vi "User Message Received.vi"(0 "Member in":refnum<class "Member.lvclass">, 5 "Message":refnum<class "Message.lvclass">, 11 "Error in":errorcluster caption="Error in (no error)") -> (4 "Member out":refnum<class "Member.lvclass">, 15 "Error out":errorcluster)   [LabVIEW 2018, in "HOG Member.lvlib" / "Member.lvclass"]
doc: "This VI runs whenever the Actor Core receives a message. Any messages not handled here are simply discarded.\n\n<B>You should not invoke the Call Parent Method node when adding this override.</B>\n\nSteen Schmidt\nGPower\n8/5 2017"
uses:
  Member.lvclass
  <vilib>/GPower/Message/Library/Message Class/Message.lvclass
  <vilib>/GPower/Message/Library/Message Class/Message.lvclass/Message.ctl
  <vilib>/GPower/Message With Data/Library/Data Message Class/Data Message.lvclass/Data Message.ctl
  Member.lvclass/Member.ctl
  1229d5d7-c008-434e-94e5-5c6cb39a25e2.vi
  <vilib>/GPower/Message With Data/Library/Data Message Class/Accessors/Get Data.vi
  <vilib>/GPower/Message With Data/Library/Data Message Class/Data Message.lvclass
  <vilib>/GPower/Dictionary - CSV/Library/Dictionary - CSV.lvlib
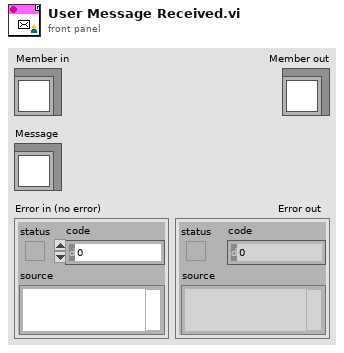
[diagram p1: front panel]
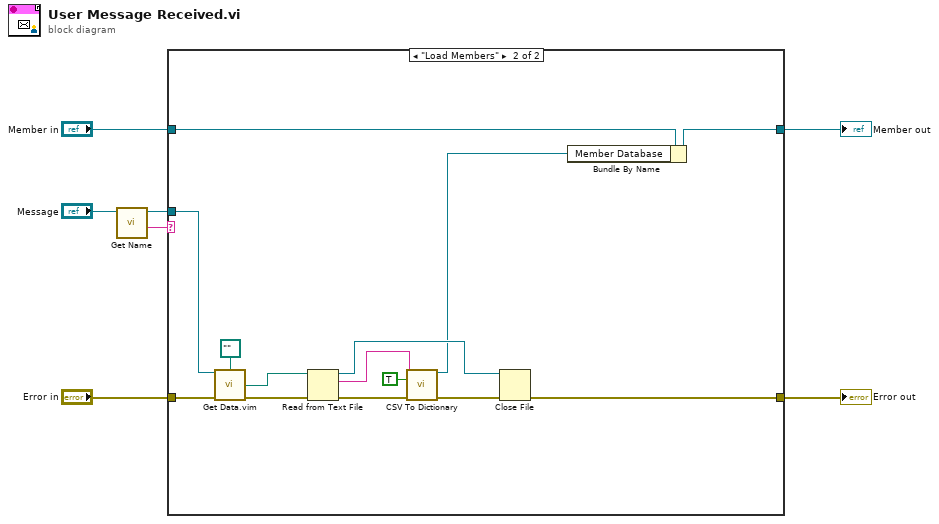
[diagram p0: block diagram]
diagram:
  n1 = call <vilib>:"Get Name.vi"("Message in"="Message") -> ("Name"=w6:string, "Message out"=w5:refnum<class "Message.lvclass">)  [unwired: 9 in]
  n2 = case shown="\"Load Members\"" w6 {
    tunnel: w5 -> [_ w23]
    tunnel: "Error in" -> [w8 w22]
    tunnel: "Member in" -> [w9 w13]
    tunnel: [w9 w11] -> w2
    tunnel: [w8 w10] -> w1
    frame "False", Default {
    }
    frame "Load Members" {
      n3 = call "Get Data.vim"("Data Message in"=w23, "Data Type"=path "", "Error in"=w22) -> ("Data"=w17:path, "Error out"=w19:errorcluster)  [unwired: 10 in, 1 out]
      n4 = Read from Text File(file (use dialog)=w17, error in=w19) -> (refnum out=w15:refnum<file>, text=w14:string, error out=w18:errorcluster)  [unwired: 2 in, 1 out]
      n5 = call <vilib>:"CSV To Dictionary.vi"("CSV String"=w14, "Header? (False)"=TRUE, "Error in"=w18) -> ("Dictionary"=w12:refnum<class "Dictionary.lvclass">, "Error out"=w16:errorcluster)  [unwired: 11 in]
      n6 = Close File(refnum=w15, error in=w16) -> (error out=w10:errorcluster)  [unwired: 1 out]
      n7 = Bundle By Name(cluster=w13, "Member Database"=w12) -> (w11:refnum<class "Member.lvclass">)
    }
  }
  "Member out" <- w2
  "Error out" <- w1
